vi "Corr Check Relative Path.vi"(8 "error in":errorcluster, 10 "root path":path, 11 "input path":path) -> (0 "error out":errorcluster, 1 "relative path valid?":bool, 2 "relative path":path, 3 "absolute path":path, 4 "input was relative?":bool)   [LabVIEW 2020]
doc: "This VI checks if input path is absolute or relative. If relative, it will try to append it to root path. It then checks file existance. It also tries to output relative path to the root no matter what type was the input path."
uses:
  <vilib>/Utility/error.llb/Error Cluster From Error Code.vi
  <vilib>/ErrorRing/Error Ring.xnode
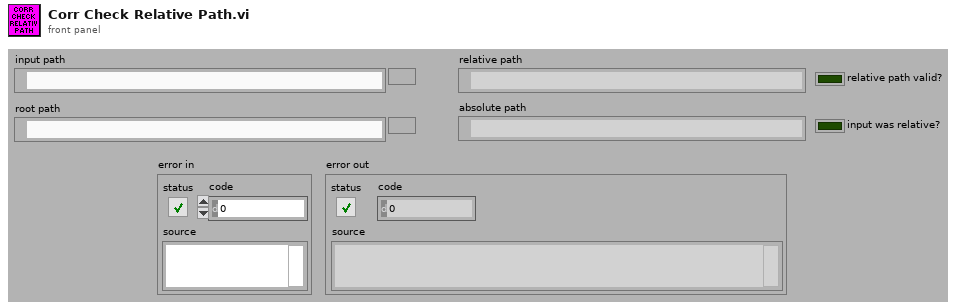
[diagram p1: front panel]
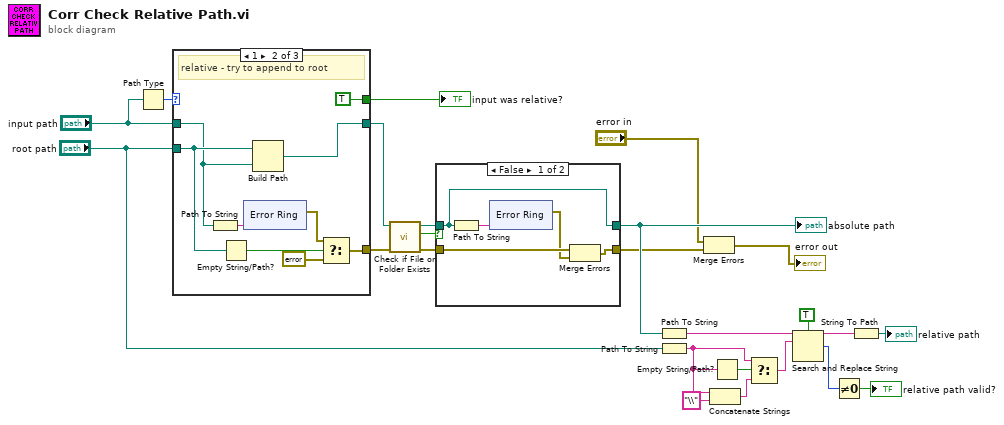
[diagram p0: block diagram]
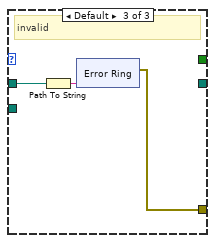
[diagram p4: hidden frame]
diagram:
  n1 = Path Type(1:"input path") -> (0:w24:i16)
  n2 = case shown="1" w24 {
    tunnel: "input path" -> [w25 w30 w43]
    tunnel: [w25 w34 _] -> w21
    tunnel: "root path" -> [_ w33 _]
    tunnel: [_ w27 w42] -> w22
    tunnel: [_ TRUE _] -> w1
    frame 0 {
      # "absolute"
    }
    frame 1 {
      # "relative - try to append to root"
      n3 = Path To String(path=w30) -> (string=w29:string)
      n4 = Empty String/Path?(string/path=w33) -> (empty?=w32:bool)
      n5 = xnode "Error Ring"("parameter 0"=w29) -> ("error out"=w31:errorcluster)
      n6 = Build Path(base path=w33, name or relative path=w30) -> (appended path=w34:path)
      n7 = Select(t=w31, s=w32, f=errorcluster {"status"=FALSE, "code"=0, "source"=""}) -> (s? t:f=w27:errorcluster)
    }
    frame Default {
      # "invalid"
      n8 = Path To String(path=w43) -> (string=w44:string)
      n9 = xnode "Error Ring"("parameter 0"=w44) -> ("error out"=w42:errorcluster)
    }
  }
  "input was relative?" <- w1
  n10 = call <vilib>:"Check if File or Folder Exists.vi"("error in (no error)"=w22, "path"=w21) -> ("error out"=w19:errorcluster, "file or folder exists?"=w20:bool, "dup path"=w18:path)  [unwired: 7 in]
  n11 = case shown="False" w20 {
    tunnel: w19 -> [w56 w63]
    tunnel: w18 -> [w52 w62]
    tunnel: [w53 w63] -> w13
    tunnel: [w52 w62] -> w14
    frame False {
      n12 = Path To String(path=w52) -> (string=w54:string)
      n13 = xnode "Error Ring"("parameter 0"=w54) -> ("error out"=w55:errorcluster)
      n14 = Merge Errors(w56, w55) -> (w53:errorcluster)
    }
    frame True {
    }
  }
  "absolute path" <- w14
  n15 = Path To String(path=w14) -> (string=w16:string)
  n16 = Path To String(path="root path") -> (string=w7:string)
  n17 = Merge Errors("error in", w13) -> (→"error out":errorcluster)
  n18 = Concatenate Strings(w7, "\\" ("string")) -> (w8:string)
  n19 = Empty String/Path?(string/path=w7) -> (empty?=w9:bool)
  n20 = Select(t=w7, s=w9, f=w8) -> (s? t:f=w5:string)
  n21 = Search and Replace String(case sensitive?=TRUE ("ignore case? (F)"), input string=w16, search string=w5) -> (result string=w10:string, number of replacements=w2:i32)  [unwired: 5 in, 2 out]
  n22 = Not Equal To 0?(x=w2) -> (x != 0?=→"relative path valid?":bool)
  n23 = String To Path(string=w10) -> (path=→"relative path":path)
